vi "Create MQTT Process.vi"(8 "error in (no error)":errorcluster, 11 "MQTT_Base in":refnum<class "MQTT_Base.lvclass">) -> (0 "error out":errorcluster, 3 "MQTT_Base out":refnum<class "MQTT_Base.lvclass">)   [LabVIEW 2013, in "MQTT Server.lvlib" / "MQTT_Base.lvclass"]
uses:
  MQTT_Base.lvclass
  Request -- cluster.ctl
  Control Packets/ControlPacket/ControlPacket.lvclass
  Response -- cluster.ctl
  MQTT_Base.lvclass/MQTT_Base.ctl
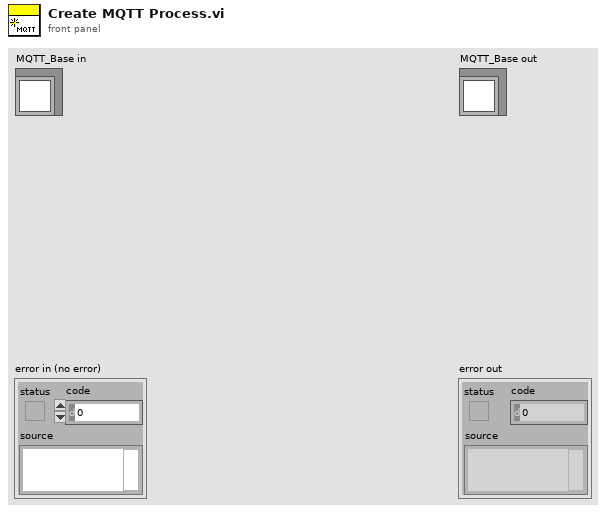
[diagram p1: front panel]
types:
  T1 = typedef "MQTT Server.lvlib/MQTT_Base.lvclass/Request -- cluster.ctl" = cluster{"RequestMsg":refnum<class "ControlPacket.lvclass">, "SessionMailbox":refnum<queue>}
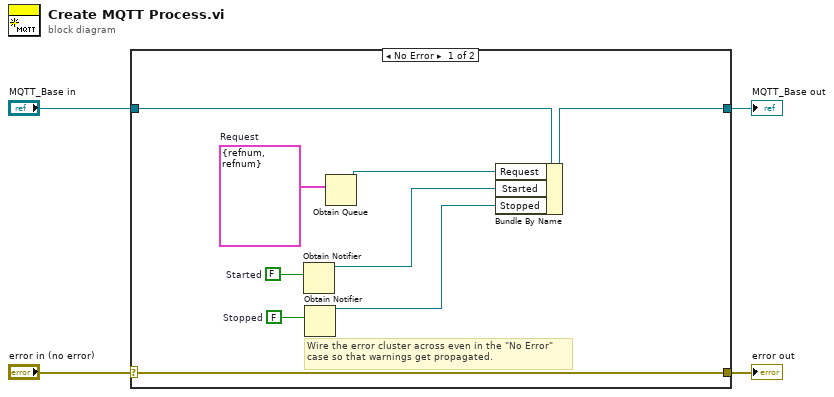
[diagram p0: block diagram]
diagram:
  n1 = case shown="No Error" "error in (no error)" {
    selector: "error in (no error)" -> [w13 w15]
    tunnel: [w13 w15] -> w3
    tunnel: [w5 w14] -> w1
    tunnel: "MQTT_Base in" -> [w6 w14]
    frame No Error {
      w10 = FALSE  # Stopped
      w11 = FALSE  # Started
      w12 = T1 {"RequestMsg"=refnum, "SessionMailbox"=refnum}  # Request
      # "Wire the error cluster across even in the \"No Error\"\ncase so that warnings get propagated."
      n2 = Obtain Notifier(notification data type=w11) -> (notifier out=w8:refnum<notifier>)  [unwired: 3 in, 2 out]
      n3 = Obtain Notifier(notification data type=w10) -> (notifier out=w7:refnum<notifier>)  [unwired: 3 in, 2 out]
      n4 = Obtain Queue(element data type=w12) -> (queue out=w9:refnum<queue>)  [unwired: 4 in, 2 out]
      n5 = Bundle By Name(cluster=w6, "Request"=w9, "Started"=w8, "Stopped"=w7) -> (w5:refnum<class "MQTT_Base.lvclass">)
    }
    frame Error {
    }
  }
  "error out" <- w3
  "MQTT_Base out" <- w1
